vi "The_Volt_Machine.vi"(1 "error in":errorcluster, 2 "Adress":string, 3 "Voltage":dbl) -> (0 "error out":errorcluster)   [LabVIEW 2010]
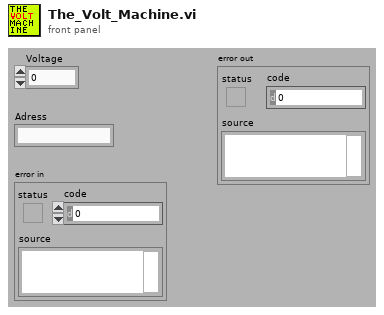
[diagram p1: front panel]
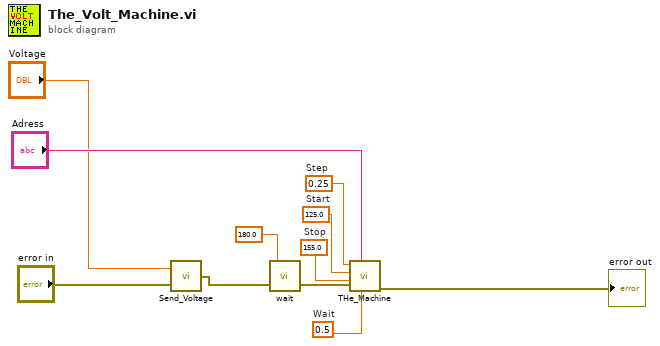
[diagram p0: block diagram]
diagram:
  w11 = 0.5  # Wait
  w9 = 155.0  # Stop
  w8 = 125.0  # Start
  w7 = 0.25  # Step
  n1 = call "Send_Voltage.vi"("error in"="error in", "Voltage"="Voltage") -> ("error out"=w3:errorcluster)
  n2 = call "wait.vi"("error in"=w3, "Wartezeit in Sek"=180.0) -> ("error out"=w10:errorcluster)  [unwired: 1 in]
  n3 = call "THe_Machine.vi"("Wait"=w11, "Adresse"="Adress", "error in (no error)"=w10, "Stop Frequency"=w9, "Start Frequency"=w8, "Stepsize"=w7) -> ("error out"=→"error out":errorcluster)  [unwired: 4 out]
